vi "Update RPC Method Template.vi"(8 "error in (no error)":errorcluster, 11 "Server Library (Library Item) in":refnum<vi>) -> (0 "error out":errorcluster, 3 "Server Library (Library Item) out":refnum<vi>)   [LabVIEW 2019, in "gRPC Scripting Tools.lvlib"]
uses:
  gRPC Scripting Tools.lvlib
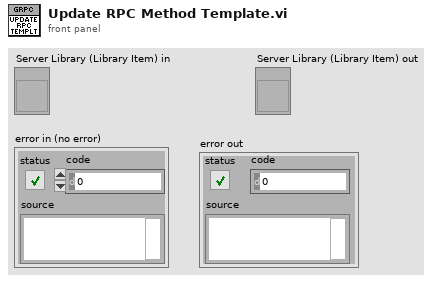
[diagram p1: front panel]
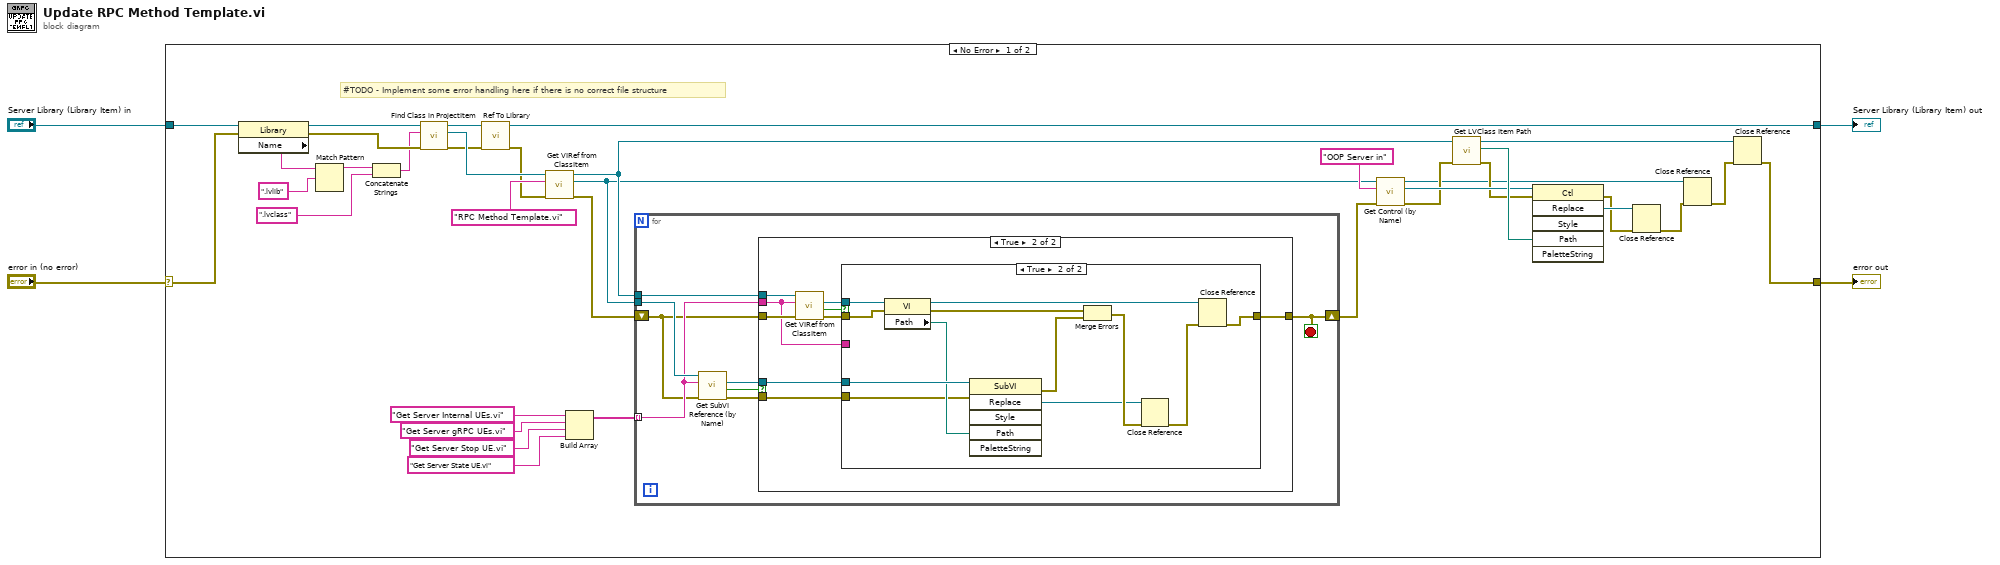
[diagram p0: block diagram]
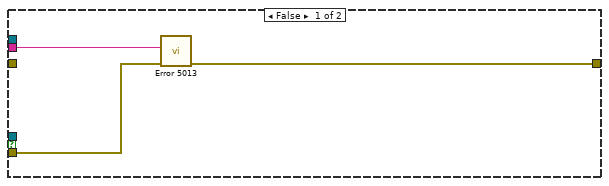
[diagram p2: hidden frame]
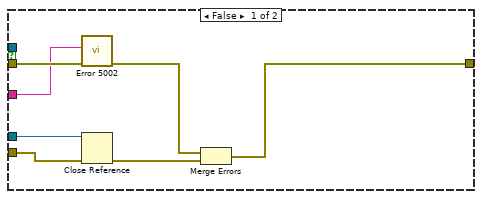
[diagram p3: hidden frame]
diagram:
  n1 = case shown="No Error" "error in (no error)" {
    selector: "error in (no error)" -> [w10 w81]
    tunnel: "Server Library (Library Item) in" -> [w28 w80]
    tunnel: [w11 w81] -> w3
    tunnel: [w8 w80] -> w1
    frame No Error {
      # "#TODO - Implement some error handling here if there is no correct file structure"
      n2 = property class="Library"(reference=w28, error in=w10) -> (reference out=w25:refnum<vi>, error out=w27:errorcluster, "Name"=w21:string)
      n3 = Match Pattern(string=w21, regular expression=".lvlib") -> (before substring=w23:string)  [unwired: 1 in, 3 out]
      n4 = Concatenate Strings(w23, ".lvclass" ("string")) -> (w26:string)
      n5 = call "Find Class in ProjectItem.vi"("error in (no error)"=w27, "Class Name"=w26, "ProjectItem in"=w25) -> ("error out"=w7:errorcluster, "LVClass out"=w30:refnum<vi>, "ProjectItem out"=w9:refnum<vi>)  [unwired: 5 in, 1 out]
      n6 = call "Ref To Library.vi"("error in (no error)"=w7, "ProjectItem in"=w9) -> ("error out"=w6:errorcluster, "Library out"=w8:refnum<vi>)  [unwired: 8 in]
      n7 = call "Get VIRef from ClassItem.vi"("error in (no error)"=w6, "Item Name"="RPC Method Template.vi", "LVClassLibrary in"=w30) -> ("error out"=w31:errorcluster, "VIref out"=w36:refnum<vi>, "LVClassLibrary out"=w39:refnum<vi>)  [unwired: 5 in, 1 out]
      n8 = Build Array("Get Server Internal UEs.vi" ("SubVI Name"), "Get Server gRPC UEs.vi" ("SubVI Name"), "Get Server Stop UE.vi" ("SubVI Name"), "Get Server State UE.vi" ("element")) -> (w35:string[])
      n9 = for {
        tunnel: w36 -> [w48]
        tunnel: w35 -> [w43] mode=indexing
        shift-right: [w45] -> w19
        shift-left: w31 -> [w41]
        tunnel: w39 -> [w42]
        stop <- w45 stop-if-true
        n10 = call "Get SubVI Reference (by Name).vi"("error in (no error)"=w41, "SubVI Name"=w43, "Owner VI in"=w48) -> ("error out"=w46:errorcluster, "Found ?"=w44:bool, "SubVI Refnum out"=w47:refnum<vi>)  [unwired: 5 in, 1 out]
        n11 = case shown="True" w44 {
          tunnel: w47 -> [_ w60]
          tunnel: w41 -> [_ w56]
          tunnel: w46 -> [w51 w59]
          tunnel: [w49 w58] -> w45
          tunnel: w42 -> [_ w57]
          tunnel: w43 -> [w50 w52]
          frame False {
            n12 = call "Error 5013.vi"("error in (no error)"=w51, "Element Name"=w50) -> ("error out"=w49:errorcluster)  [unwired: 9 in]
          }
          frame True {
            n13 = call "Get VIRef from ClassItem.vi"("error in (no error)"=w56, "Item Name"=w52, "LVClassLibrary in"=w57) -> ("error out"=w54:errorcluster, "Found ?"=w53:bool, "VIref out"=w55:refnum<vi>)  [unwired: 5 in, 1 out]
            n14 = case shown="True" w53 {
              tunnel: w60 -> [w67 w79]
              tunnel: w59 -> [w66 w77]
              tunnel: [w64 w71] -> w58
              tunnel: w55 -> [_ w69]
              tunnel: w54 -> [w63 w68]
              tunnel: w52 -> [w62 _]
              frame False {
                n15 = call "Error 5002.vi"("error in (no error)"=w63, "Method Name"=w62) -> ("error out"=w61:errorcluster)  [unwired: 9 in]
                n16 = Close Reference(reference=w67, error in (no error)=w66) -> (error out=w65:errorcluster)
                n17 = Merge Errors(w61, w65) -> (w64:errorcluster)
              }
              frame True {
                n18 = property class="VI"(reference=w69, error in=w68) -> (reference out=w72:refnum<vi>, error out=w75:errorcluster, "Path"=w78:path)
                n19 = invoke class="SubVI" method="Replace"(reference=w79, error in=w77, "Path"=w78) -> (error out=w76:errorcluster, "Replace"=w73:refnum<vi>)  [unwired: 3 in, 4 out]
                n20 = Merge Errors(w75, w76) -> (w74:errorcluster)
                n21 = Close Reference(reference=w73, error in (no error)=w74) -> (error out=w70:errorcluster)
                n22 = Close Reference(reference=w72, error in (no error)=w70) -> (error out=w71:errorcluster)
              }
            }
          }
        }
      }
      n23 = call "Get Control (by Name).vi"("error in (no error)"=w19, "Control Label"="OOP Server in" ("Constant Label"), "Owner VI in"=w36) -> ("error out"=w20:errorcluster, "Control Refnum"=w38:refnum<vi>, "Owner VI out"=w14:refnum<vi>)  [unwired: 5 in, 1 out]
      n24 = call "Get LVClass Item Path.vi"("error in (no error)"=w20, "LVClassLibrary in"=w39) -> ("error out"=w18:errorcluster, "Path"=w40:path, "LVClassLibrary out"=w13:refnum<vi>)  [unwired: 7 in]
      n25 = invoke class="Ctl" method="Replace"(reference=w38, error in=w18, "Path"=w40) -> (error out=w16:errorcluster, "Replace"=w17:refnum<vi>)  [unwired: 3 in, 4 out]
      n26 = Close Reference(reference=w17, error in (no error)=w16) -> (error out=w15:errorcluster)
      n27 = Close Reference(reference=w14, error in (no error)=w15) -> (error out=w12:errorcluster)
      n28 = Close Reference(reference=w13, error in (no error)=w12) -> (error out=w11:errorcluster)
    }
    frame Error {
    }
  }
  "error out" <- w3
  "Server Library (Library Item) out" <- w1
